vi "Get Component Settings.vi"(8 "error in (no error)":errorcluster, 10 "settings id":T2, 11 "Item Ref in":T1 format="%.0x") -> (0 "error out":errorcluster, 2 "component settings":T3[](array[typedef]), 3 "Item Ref out":T1 format="%.0x")   [LabVIEW 2017, in "DSF System Explorer.lvlib"]
uses:
  DSF System Explorer.lvlib
  DSF Core.lvlibp/Typedefs/DSF Settings Info.ctl
  DSF Core.lvlibp/Typedefs/DSF Version Info.ctl
  DSF Core.lvlibp/Typedefs/DSF Configuration ID.ctl
  <vilib>/NI Veristand/Custom Device API/Custom Device Item Ref.ctl
  DSF Core.lvlibp
  <vilib>/NI Veristand/Custom Device API/Custom Device API.lvlib
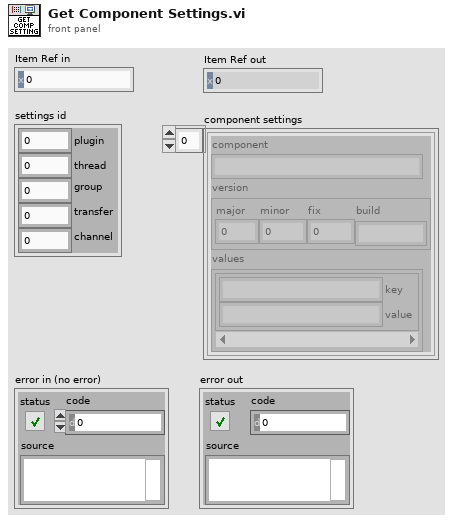
[diagram p1: front panel]
types:
  T1 = typedef "Custom Device API.lvlib/Custom Device Item Ref.ctl" = u64
  T2 = typedef "DSF Core.lvlibp/DSF Configuration ID.ctl" = cluster{"plugin":i32, "thread":i32, "group":i32, "transfer":i32, "channel":i32}
  T3 = typedef "DSF Core.lvlibp/DSF Settings Info.ctl" = cluster{"component":string, "version":T4, "values":cluster{"key":string, "value":string}[]}
  T4 = typedef "DSF Core.lvlibp/DSF Version Info.ctl" = cluster{"major":u32, "minor":u32, "fix":u32, "build":string}
  T5 = typedef "DSF Core.lvlibp/DSF Engine Framework Configuration.ctl" = cluster{"plugins":T6[]}
  T6 = typedef "DSF Core.lvlibp/DSF Engine Plugin Configuration.ctl" = cluster{"core":T7, "component settings":T3[], "threads":T9[]}
  T7 = typedef "DSF Core.lvlibp/DSF Core Plugin Configuration.ctl" = cluster{"name":string, "components":string[], "cycle timing":T8}
  T8 = typedef "DSF Core.lvlibp/DSF Timing Info.ctl" = cluster{"priority":u64, "decimation":u64, "offset":u64}
  T9 = typedef "DSF Core.lvlibp/DSF Engine Plugin Thread Configuration.ctl" = cluster{"core":T10, "component settings":T3[], "transfer groups":T11[]}
  T10 = typedef "DSF Core.lvlibp/DSF Core Thread Configuration.ctl" = cluster{"processor":i32, "priority offset":i16}
  T11 = typedef "DSF Core.lvlibp/DSF Engine Transfer Group Configuration.ctl" = cluster{"core":T12, "component settings":T3[], "transfers":T15[]}
  T12 = typedef "DSF Core.lvlibp/DSF Core Group Configuration.ctl" = cluster{"name":string, "direction":T13, "cycle timing":T8, "timeout behavior":T14}
  T13 = typedef "DSF Core.lvlibp/DSF Direction.ctl" = enum8{"Tx", "Rx"}
  T14 = typedef "DSF Core.lvlibp/DSF Timeout Behavior.ctl" = enum8{"Increment Late Count", "Throw Error"}
  T15 = typedef "DSF Core.lvlibp/DSF Engine Transfer Configuration.ctl" = cluster{"core":T16, "component settings":T3[], "channels":T17[]}
  T16 = typedef "DSF Core.lvlibp/DSF Core Transfer Configuration.ctl" = cluster{"name":string}
  T17 = typedef "DSF Core.lvlibp/DSF Engine Channel Configuration.ctl" = cluster{"core":T18, "component settings":T3[]}
  T18 = typedef "DSF Core.lvlibp/DSF Core Channel Configuration.ctl" = cluster{"name":string, "units":string, "engine data type":T19, "string data type":T19, "string offset":u64}
  T19 = typedef "DSF Core.lvlibp/DSF Data Type.ctl" = enum8{"Bool", "SGL", "DBL", "I8", "I16", "I32", "I64", "U8", "U16", "U32", "U64"}
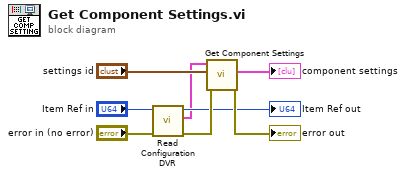
[diagram p0: block diagram]
diagram:
  n1 = call "Read Configuration DVR.vi"("error in (no error)"="error in (no error)", "Item Ref in"="Item Ref in") -> ("error out"=w6:errorcluster, "framework configuration"=w1:T5, "Item Ref out"=→"Item Ref out":T1)  [unwired: 7 in]
  n2 = call "Get Component Settings.vi"("error in (no error)"=w6, "settings id"="settings id", "framework configuration in"=w1) -> ("error out"=→"error out":errorcluster, "component settings"=→"component settings":T3[])  [unwired: 6 in, 1 out]
